vi "Check Unknown.vi"(8 "error in (no error)":errorcluster, 9 "Known Found?":bool, 10 "filenames":string[](array[string]), 11 "Working Dir":path) -> (0 "error out":errorcluster, 1 "Abort?":bool, 3 "Working Dir Out":path, 4 "Tags Removed":string[](array[string]))   [LabVIEW 2024]
uses:
  TypeDefs/Tag Cmd.ctl
  <userlib>/_OpenG.lib/file/file.llb/Strip Path Extension - String__ogtk.vi
  <userlib>/_OpenG.lib/file/file.llb/openg_file.lvlib
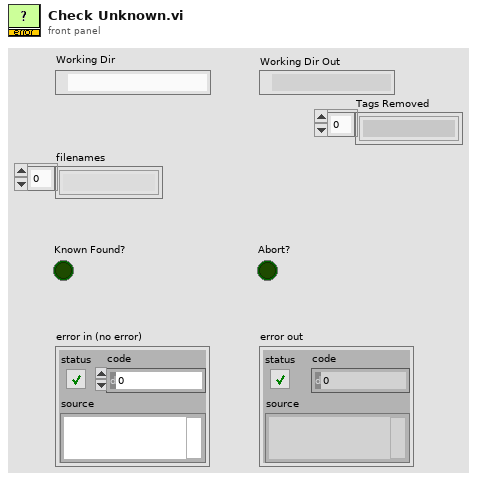
[diagram p1: front panel]
types:
  T1 = typedef "Tag Cmd.ctl" = enum16{"Init", "Get Known", "Set Known"}
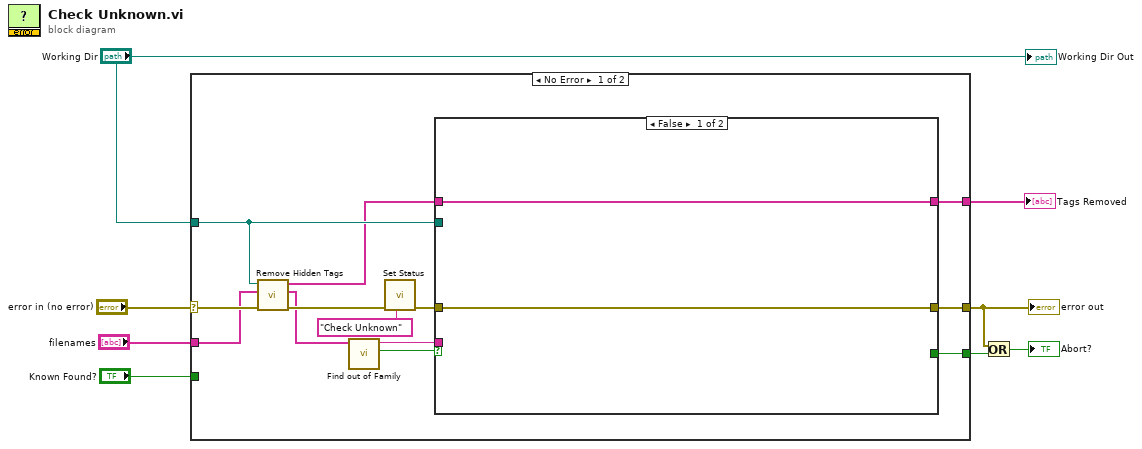
[diagram p0: block diagram]
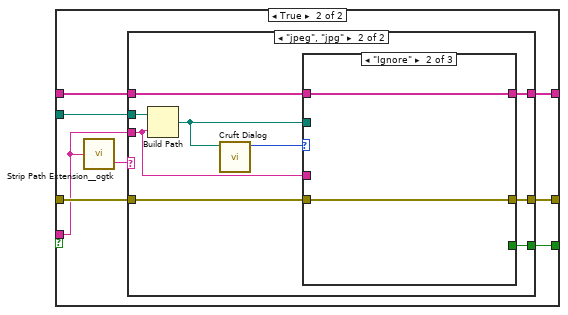
[diagram p2: hidden frame]
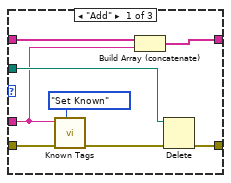
[diagram p4: hidden frame]
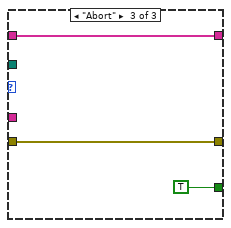
[diagram p5: hidden frame]
diagram:
  n1 = case shown="No Error" "error in (no error)" {
    selector: "error in (no error)" -> [w14 w56]
    tunnel: "Known Found?" -> [_ _]
    tunnel: [w21 w56] -> w3
    tunnel: "filenames" -> [w11 _]
    tunnel: "Working Dir" -> [w12 _]
    tunnel: [w20 _] -> w4
    tunnel: [w17 _] -> w1
    frame No Error {
      n2 = call "Remove Hidden Tags.vi"("error in (no error)"=w14, "filenames"=w11, "Working Dir"=w12) -> ("error out"=w13:errorcluster, "filenames out"=w9:string[], "Tag Name"=w10:string[])  [unwired: 6 in]
      n3 = call "Find out of Family.vi"("filenames"=w9) -> ("Found"=w16:bool, "Out of Family"=w15:string)  [unwired: 9 in]
      n4 = call "Set Status.vi"("Status Message"="Check Unknown" ("Value"), "error in (no error)"=w13) -> ("error out"=w19:errorcluster)  [unwired: 9 in]
      n5 = case shown="False" w16 {
        tunnel: [w23 w31] -> w21
        tunnel: w19 -> [w23 w29]
        tunnel: w12 -> [_ w28]
        tunnel: [_ w30] -> w20
        tunnel: [w22 w26] -> w17
        tunnel: w15 -> [_ w25]
        tunnel: w10 -> [w22 w24]
        frame False {
        }
        frame True {
          n6 = call-poly <userlib>:"Strip Path Extension__ogtk.vi"("path"=w25) -> ("extension"=w27:string)  [unwired: 1 out]
          n7 = case shown="\"jpeg\", \"jpg\"" w27 {
            tunnel: [w33 w42] -> w31
            tunnel: [_ w41] -> w30
            tunnel: w29 -> [w33 w40]
            tunnel: w28 -> [_ w39]
            tunnel: [w32 w36] -> w26
            tunnel: w25 -> [_ w35]
            tunnel: w24 -> [w32 w34]
            frame Default {
            }
            frame "jpeg", "jpg" {
              n8 = Build Path(base path=w39, name or relative path=w35) -> (appended path=w38:path)
              n9 = call "Cruft Dialog.vi"("Path"=w38) -> ("Result"=w37:enum16{"Add", "Ignore", "Abort"})  [unwired: 10 in]
              n10 = case shown="\"Ignore\"" w37 {
                tunnel: w40 -> [w50 w52 w55]
                tunnel: w35 -> [w44 _ _]
                tunnel: [w47 w52 w55] -> w42
                tunnel: [_ _ TRUE] -> w41
                tunnel: w38 -> [w46 _ _]
                tunnel: [w43 w51 w53] -> w36
                tunnel: w34 -> [w45 w51 w53]
                frame "Add" {
                  n11 = call "Known Tags.vi"("Tag Cmd"=Tag_Cmd."Set Known", "error in (no error)"=w50, "New Tag"=w44) -> ("error out"=w49:errorcluster)  [unwired: 7 in, 1 out]
                  n12 = Build Array (concatenate)(w45, w44) -> (w43:string[])
                  n13 = Delete(path (use dialog)=w46, error in=w49) -> (error out=w47:errorcluster)  [unwired: 3 in, 2 out]
                }
                frame "Ignore" {
                }
                frame "Abort" {
                }
              }
            }
          }
        }
      }
    }
    frame Error {
    }
  }
  "error out" <- w3
  "Tags Removed" <- w1
  n14 = Or(x=w3, y=w4) -> (x .or. y?=→"Abort?":bool)
  "Working Dir Out" <- "Working Dir"
